vi "SDCP - Standard Message Frames Editor - Generate Transmit Code.vi"(2 "error in (no error)":errorcluster, 3 "Frame details":T2(array[cluster]), 4 "Transmit tick (us)":dbl) -> (0 "error out":errorcluster, 1 "Output":string)   [LabVIEW 2020]
uses:
  Typedefs/SDCP - Standard Message Frames Editor - Parameter cluster.ctl
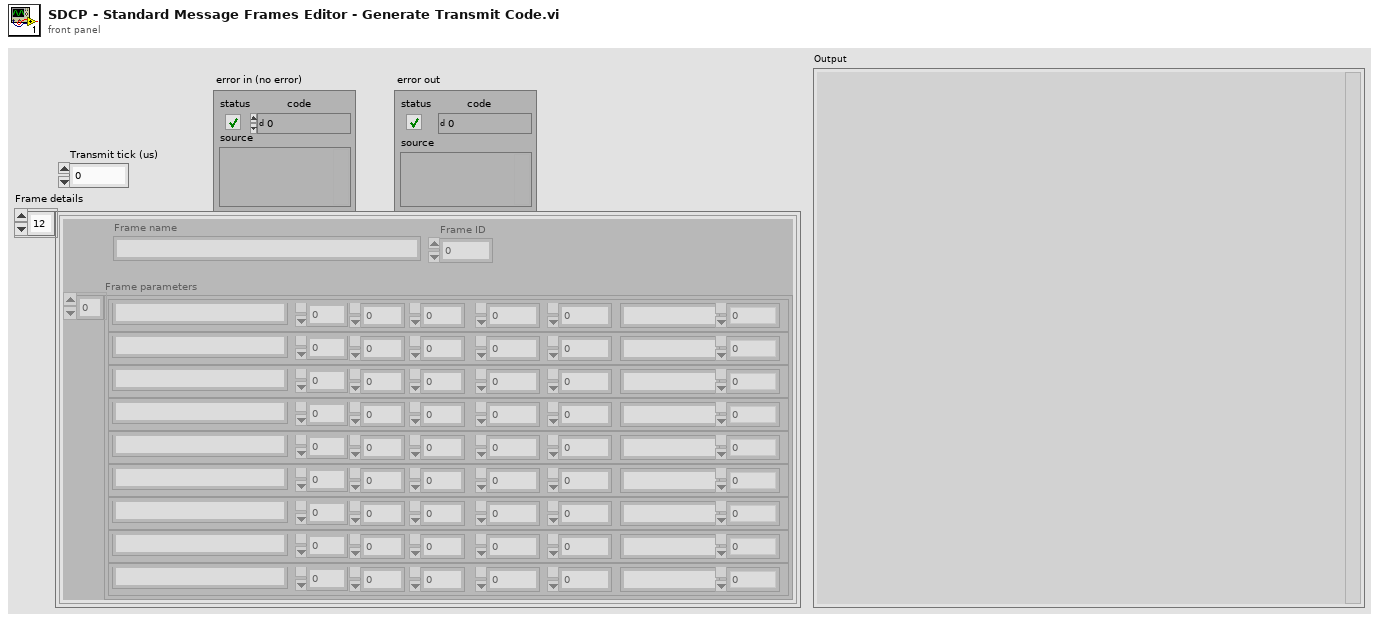
[diagram p1: front panel]
types:
  T1 = typedef "SDCP - Standard Message Frames Editor - Parameter cluster.ctl" = cluster{"Parameter name":string, "Start Bit":i32, "Stop Bit":i32, "Length":i32, "Factor":dbl, "Offset":dbl, "Data type":string, "Cycle time":dbl}
  T2 = cluster{"Frame name":string, "Frame ID":i32, "Frame parameters":T1[]}[]
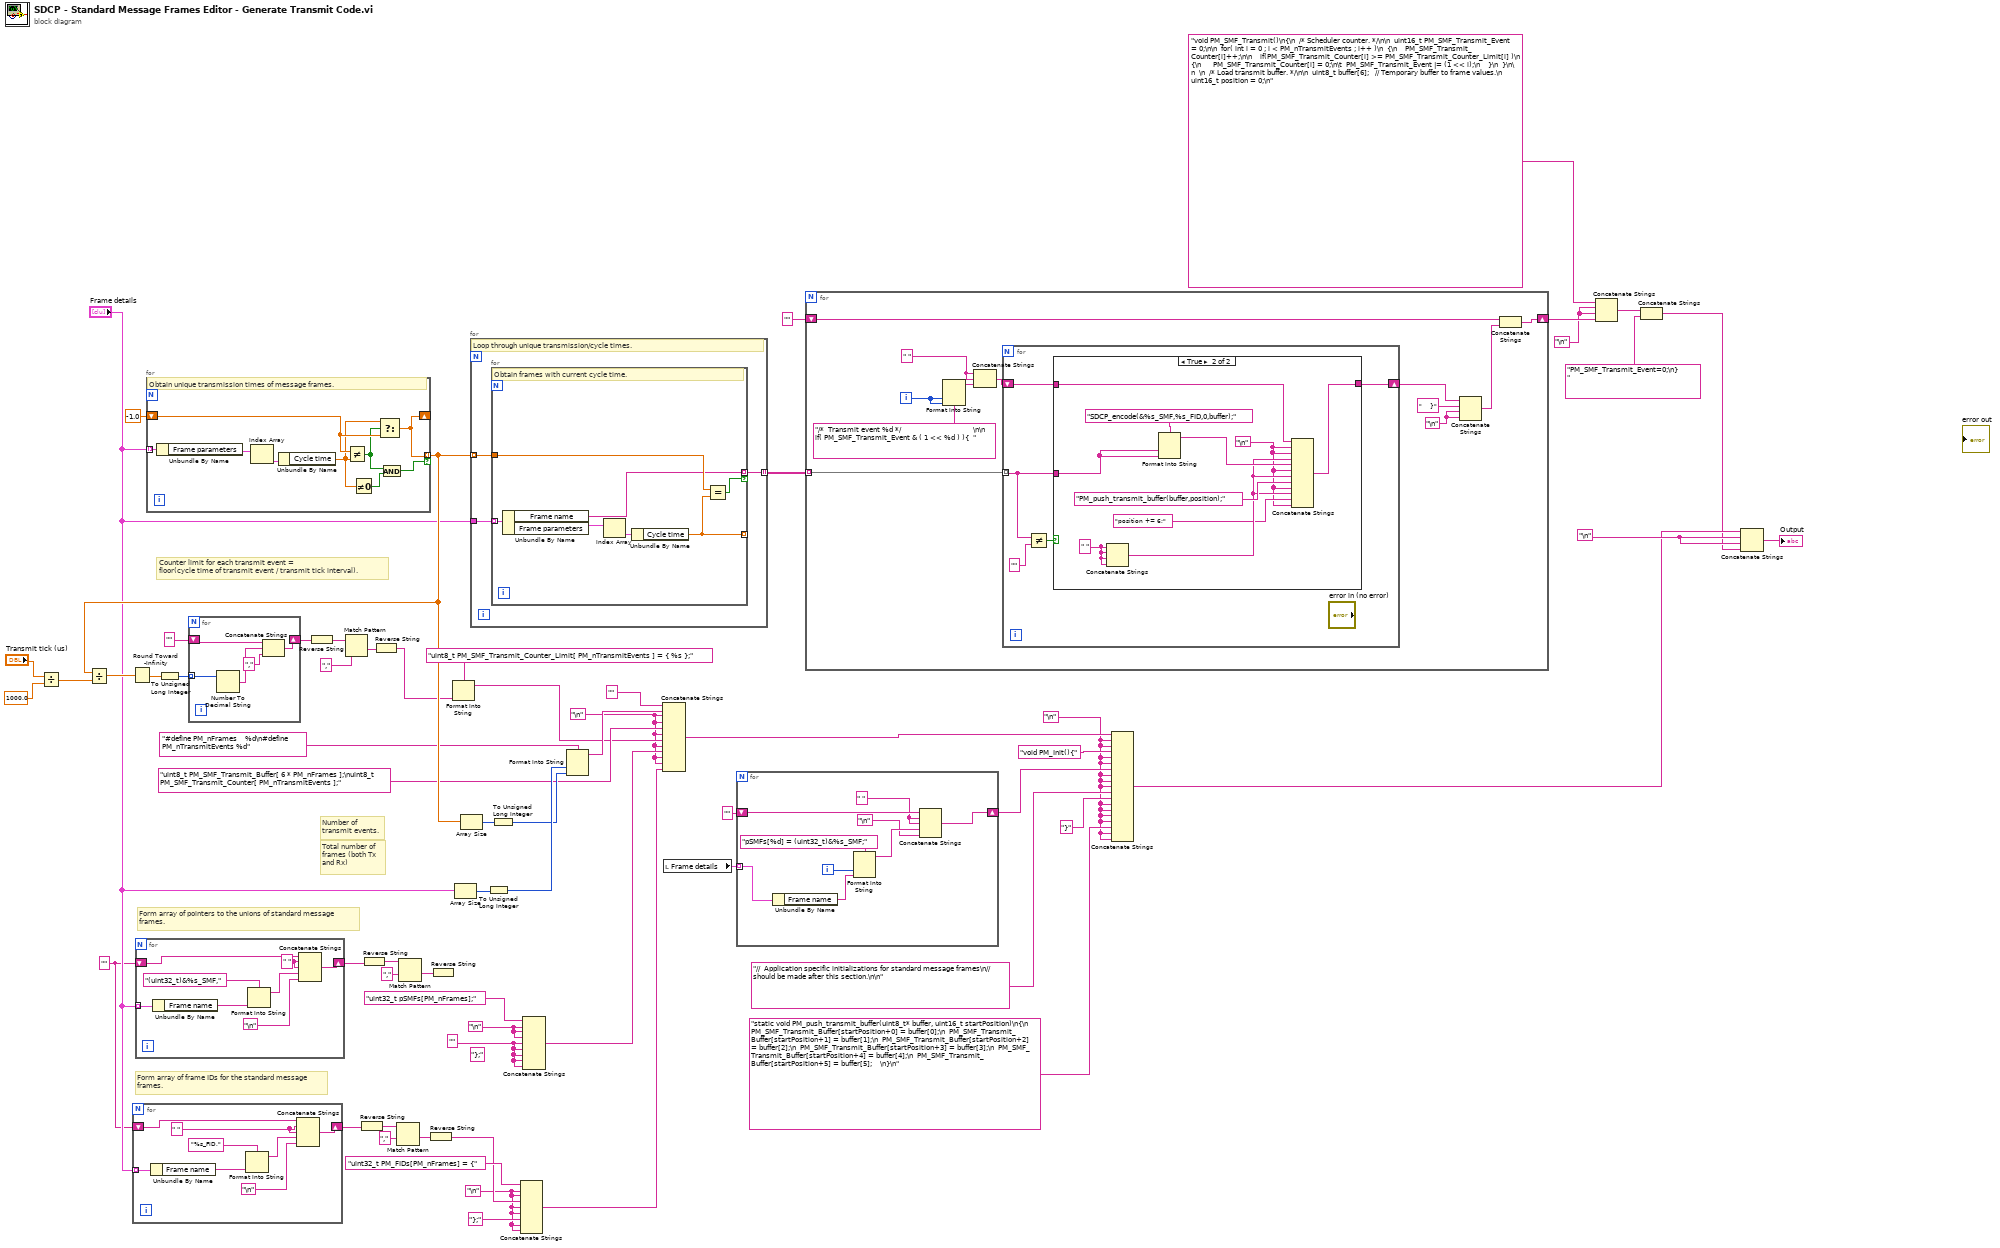
[diagram p0: block diagram]
diagram:
  w18 = "\n"
  w22 = "\n"
  w11 = "\n"
  w33 = ""
  w37 = "\n"
  (unwired) "};" ("string")
  w34 = "\n"
  w13 = ""
  w1 = "\n"
  # "Form array of frame IDs for the standard message\nframes."
  # "Form array of pointers to the unions of standard message\nframes."
  # "Total number of\nframes (both Tx\nand Rx)"
  # "Number of \ntransmit events."
  # "Counter limit for each transmit event = \nfloor(cycle time of transmit event / transmit tick interval)."
  n1 = Divide(x="Transmit tick (us)", y=1000.0) -> (x/y=w61:dbl)
  n2 = for {
    tunnel: "Frame details" -> [w72] mode=indexing
    shift-right: [w69] -> w44
    shift-left: w13 -> [w68]
    w65 = " "
    n3 = Unbundle By Name(w72) -> ("Frame name"=w70:string)
    n4 = Format Into String(format string="%s_FID,", w70) -> (resulting string=w66:string)  [unwired: 2 in, 1 out]
    n5 = Concatenate Strings(w68, w65, w65, w66, "\n") -> (w69:string)
  }
  n6 = for {
    tunnel: "Frame details" -> [w80] mode=indexing
    shift-right: [w77] -> w50
    shift-left: w13 -> [w76]
    w73 = " " ("string")
    n7 = Unbundle By Name(w80) -> ("Frame name"=w78:string)
    n8 = Format Into String(format string="(uint32_t)&%s_SMF,", w78) -> (resulting string=w74:string)  [unwired: 2 in, 1 out]
    n9 = Concatenate Strings(w76, w73, w73, w74, "\n") -> (w77:string)
  }
  n10 = for {
    tunnel: [w89] -> _ mode=indexing
    tunnel: "Frame details" -> [w89] mode=indexing
    shift-right: [w85] -> _
    shift-left: -1.0 -> [w86]
    tunnel: [w85] -> w58 mode=indexing if=w81
    # "Obtain unique transmission times of message frames."
    n11 = Unbundle By Name(w89) -> ("Frame parameters"=w88:T1[])
    n12 = Index Array(array=w88) -> (element=w87:T1)  [unwired: 1 in]
    n13 = Unbundle By Name(w87) -> ("Cycle time"=w84:dbl)
    n14 = Not Equal?(x=w86, y=w84) -> (x != y?=w82:bool)
    n15 = Not Equal To 0?(x=w84) -> (x != 0?=w83:bool)
    n16 = Select(t=w84, s=w82, f=w86) -> (s? t:f=w85:dbl)
    n17 = And(x=w82, y=w83) -> (x .and. y?=w81:bool)
  }
  n18 = Divide(x=w58, y=w61) -> (x/y=w60:dbl[])
  n19 = Round Toward -Infinity(1:w60) -> (0:w59:dbl[])
  n20 = To Unsigned Long Integer(number=w59) -> (unsigned 32bit integer=w10:u32[])
  n21 = for {
    tunnel: w10 -> [w94] mode=indexing
    shift-right: [w91] -> w8
    shift-left: "" -> [w93]
    n22 = Number To Decimal String(number=w94) -> (decimal integer string=w92:string)  [unwired: 1 in]
    n23 = Concatenate Strings(w93, w92, "," ("string")) -> (w91:string)
  }
  n24 = Reverse String(1:w8) -> (0:w7:string)
  n25 = Match Pattern(string=w7, regular expression=",") -> (after substring=w6:string)  [unwired: 1 in, 3 out]
  n26 = Reverse String(1:w44) -> (0:w43:string)
  n27 = Reverse String(1:w50) -> (0:w49:string)
  n28 = Reverse String(1:w6) -> (0:w5:string)
  n29 = Match Pattern(string=w43, regular expression=",") -> (after substring=w41:string)  [unwired: 1 in, 3 out]
  n30 = Match Pattern(string=w49, regular expression=",") -> (after substring=w47:string)  [unwired: 1 in, 3 out]
  n31 = Reverse String(1:w41) -> (0:w39:string)
  n32 = Reverse String(1:w47) -> ()  [unwired: 1 out]
  n33 = Format Into String(format string="uint8_t PM_SMF_Transmit_Counter_Limit[ PM_nTransmitEvents ] = { %s };", w5) -> (resulting string=w2:string)  [unwired: 2 in, 1 out]
  n34 = Array Size(array="Frame details") -> (size(s)=w56:i32)
  n35 = Array Size(array=w58) -> (size(s)=w57:i32)
  n36 = for {
    tunnel: w58 -> [w97] mode=indexing
    tunnel: "Frame details" -> [w96]
    tunnel: [w95] -> w25 mode=indexing
    # "Loop through unique transmission/cycle times."
    n37 = for {
      tunnel: w97 -> [w101]
      tunnel: w96 -> [w104] mode=indexing
      tunnel: [w100] -> w95 mode=indexing if=w99
      tunnel: [w98] -> _ mode=indexing
      # "Obtain frames with current cycle time."
      n38 = Unbundle By Name(w104) -> ("Frame name"=w100:string, "Frame parameters"=w103:T1[])
      n39 = Index Array(array=w103) -> (element=w102:T1)  [unwired: 1 in]
      n40 = Unbundle By Name(w102) -> ("Cycle time"=w98:dbl)
      n41 = Equal?(x=w101, y=w98) -> (x = y?=w99:bool)
    }
  }
  n42 = To Unsigned Long Integer(number=w56) -> (unsigned 32bit integer=w54:u32)
  n43 = To Unsigned Long Integer(number=w57) -> (unsigned 32bit integer=w53:u32)
  n44 = Concatenate Strings("uint32_t PM_FIDs[PM_nFrames] = {" ("string"), w37, w37, w39, w37, w37, "};" ("string"), w37, w37) -> (w35:string)
  n45 = Concatenate Strings("uint32_t pSMFs[PM_nFrames];" ("string"), w34, w34, w34, w33, w33, w33, w33, w33) -> (w45:string)
  n46 = Format Into String(format string="#define PM_nFrames    %d\n#define PM_nTransmitEvents %d", w54, w53) -> (resulting string=w52:string)  [unwired: 2 in, 1 out]
  n47 = Concatenate Strings("" ("string"), w52, w1, w1, "uint8_t PM_SMF_Transmit_Buffer[ 6 * PM_nFrames ];\nuint8_t PM_SMF_Transmit_Counter[ PM_nTransmitEvents ];", w1, w2, w1, w45, w1, w1, w35) -> (w32:string)
  n48 = local read "Frame details"() -> (w30:T2)
  n49 = for {
    tunnel: w30 -> [w112] mode=indexing
    shift-right: [w106] -> w28
    shift-left: "" -> [w109]
    i -> [w110]
    w105 = " "
    n50 = Unbundle By Name(w112) -> ("Frame name"=w111:string)
    n51 = Format Into String(format string="pSMFs[%d] = (uint32_t)&%s_SMF;", w110, w111) -> (resulting string=w108:string)  [unwired: 2 in, 1 out]
    n52 = Concatenate Strings(w109, w105, w105, w108, "\n") -> (w106:string)
  }
  n53 = for {
    tunnel: w25 -> [w124] mode=indexing
    shift-right: [w119] -> w23
    shift-left: "" -> [w121]
    i -> [w116]
    w114 = " "
    w120 = "\n"
    n54 = Format Into String(format string="/*  Transmit event %d */                                    \n\n  if( PM_SMF_Transmit_Event & ( 1 << %d ) ){  ", w116, w116) -> (resulting string=w118:string)  [unwired: 2 in, 1 out]
    n55 = Concatenate Strings(w114, w114, w118) -> (w117:string)
    n56 = for {
      shift-right: [w130] -> w123
      shift-left: w117 -> [w129]
      tunnel: w124 -> [w127] mode=indexing
      n57 = Not Equal?(x=w127, y="") -> (x != y?=w128:bool)
      n58 = case shown="True" w128 {
        tunnel: [w131 w140] -> w130
        tunnel: w127 -> [_ w139]
        tunnel: w129 -> [w131 w138]
        frame False {
        }
        frame True {
          w132 = " " ("string")
          w133 = "\n"
          n59 = Concatenate Strings(w132, w132, w132, w132) -> (w135:string)
          n60 = Format Into String(format string="SDCP_encode(&%s_SMF,%s_FID,0,buffer);", w139, w139) -> (resulting string=w137:string)  [unwired: 2 in, 1 out]
          n61 = Concatenate Strings(w138, w133, w133, w135, w137, w133, w135, "PM_push_transmit_buffer(buffer,position);" ("string"), w133, w135, "position += 6;", w133) -> (w140:string)
        }
      }
    }
    n62 = Concatenate Strings(w123, "    }" ("string"), w120, w120) -> (w115:string)
    n63 = Concatenate Strings(w121, w115) -> (w119:string)
  }
  n64 = Concatenate Strings(w32, w11, w11, "void PM_Init(){" ("string"), w11, w11, w28, w11, w11, w11, "//  Application specific initializations for standard message frames\n//  should be made after this section.\n\n", "}", w11, w11, w11, w11, "static void PM_push_transmit_buffer(uint8_t* buffer, uint16_t startPosition)\n{\n  PM_SMF_Transmit_Buffer[startPosition+0] = buffer[0];\n  PM_SMF_Transmit_Buffer[startPosition+1] = buffer[1];\n  PM_SMF_Transmit_Buffer[startPosition+2] = buffer[2];\n  PM_SMF_Transmit_Buffer[startPosition+3] = buffer[3];\n  PM_SMF_Transmit_Buffer[startPosition+4] = buffer[4];\n  PM_SMF_Transmit_Buffer[startPosition+5] = buffer[5];    \n}\n", w11, w11) -> (w17:string)
  n65 = Concatenate Strings("void PM_SMF_Transmit()\n{\n  /* Scheduler counter. */\n\n  uint16_t PM_SMF_Transmit_Event = 0;\n\n  for( int i = 0 ; i < PM_nTransmitEvents ; i++ )\n  {\n    PM_SMF_Transmit_Counter[i]++;\n\n    if(PM_SMF_Transmit_Counter[i] >= PM_SMF_Transmit_Counter_Limit[i] )\n    {\n      PM_SMF_Transmit_Counter[i] = 0;\n\t  PM_SMF_Transmit_Event |= (1 << i);\n    }\n  }\n\n  \n  /* Load transmit buffer. */\n\n  uint8_t buffer[6];   // Temporary buffer to frame values.\n  uint16_t position = 0;\n", w22, w22, w23) -> (w20:string)
  n66 = Concatenate Strings(w20, "PM_SMF_Transmit_Event=0;\n}                                                          " ("string")) -> (w16:string)
  n67 = Concatenate Strings(w17, w18, w18, w16) -> (→"Output":string)
